vi "Handle Double Click on Element.vi"(8 "error in (no error)":errorcluster, 10 "Unique ID":string, 11 "Process Builder Model in":refnum<class "Process Builder Model.lvclass">) -> (0 "error out":errorcluster, 3 "Process Builder Model out":refnum<class "Process Builder Model.lvclass">)   [LabVIEW 2019, in "Process Builder Model.lvclass"]
uses:
  <vilib>/gpm_packages/@cs/Car-wash/Source/Process Builder Model/Process Builder Model.lvclass
  <vilib>/gpm_packages/@cs/Test-executive-builder/Source/Test Executive Builder Model/Test Executive Builder Model/Test Executive Builder Model.lvclass
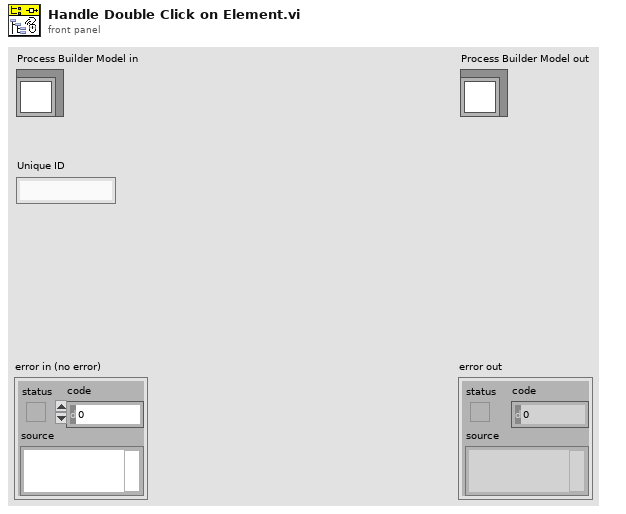
[diagram p1: front panel]
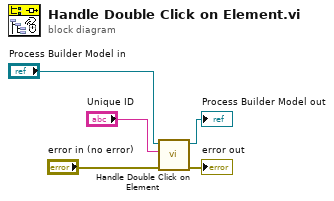
[diagram p0: block diagram]
diagram:
  n1 = call-parent "Handle Double Click on Element.vi"("error in (no error)"="error in (no error)", "Unique ID"="Unique ID", "Test Executive Builder Model in"="Process Builder Model in") -> ("error out"=→"error out":errorcluster, "Test Executive Builder Model out"=→"Process Builder Model out":refnum<class "Process Builder Model.lvclass">)  [unwired: 7 in]
